vi "LED_control.vi"() -> ()   [LabVIEW 2018]
uses:
  <instrlib>/niDMM/nidmm.llb/niDMM Function.ctl
  <instrlib>/niDMM/nidmm.llb/niDMM Resolution in Digits.ctl
  <instrlib>/niDCPower/nidcpower.llb/niDCPower Measurement Type.ctl
  <instrlib>/niDMM/nidmm.llb/niDMM Configure Measurement Digits.vi
  <vilib>/Instr/_visa.llb/VISA Configure Serial Port (Instr).vi
panel:
  in  "Command":string="led_on"
  in  "Записать":bool
  in  "Tab Control":enum32{"Рабочая область", "Служебная область"}(tab)
  out "Тип индикатора":string
  in  "Питание":bool
  in  "Стоп":bool
  in  "Resource Name":refnum<k15>="PXI1Slot2" caption="Источник питания"
  in  "Мультиметр":refnum<k15>="PXI1Slot3" caption="NI DMM 1"
  in  "V_MB, V":dbl=6.0 caption="voltage level" format="%_6p"
  in  "curlim_V_MB, A":dbl=0.3 caption="current limit" format="%_6p"
  in  "curlim_V_RESERVE, A":dbl=0.1 caption="current limit" format="%_6p"
  out "currentmes_V_MB, A":dbl caption="measurement" format="%_6g"
  out "currentmes_V_RESERVE, A":dbl caption="measurement" format="%_6g"
  in  "V_RESERVE, V":dbl caption="voltage level" format="%_6p"
  out "chart_2":dbl(graph)=8.556104343922883e-07
  out "chart_0":dbl(graph)=5.42616690347781e-05 caption="Waveform Chart 5"
  in  "curlim_V_LED, A":dbl=0.01999999999999985 caption="current limit" format="%_6p"
  in  "V_LED, V":dbl=1.7000000000000006 caption="voltage level" format="%_6p"
  out "chart_1":dbl(graph)=2.456762028615791e-06 caption="Waveform Chart 5"
  out "currentmes_V_LED, A":dbl caption="measurement" format="%_6g"
  in  "NI DMM 1 Current Range 3":string(combo)="0,1" caption="Range"
  out "Real Current, А":dbl=1.3612861948786303e-08 format="%.5f"
  in  "NI DMM 1 units 3":string(combo)="1000" caption="Units"
  out "NI DMM 1 Current Char 3":dbl(graph)=0.013612861948786303
  out "NI DMM 1 Current 3":dbl caption="Current" format="%_6g"
  in  "Arduino":refnum<visa-resource-name>="COM5"
  in  "Сегменты":bool[](array[boolean])=[FALSE, FALSE, FALSE, FALSE, FALSE, FALSE, FALSE, FALSE, FALSE, FALSE]
  out "Разряд":dbl
  out "+/-":bool
  out "Power off":bool
  # "необходимо выдерживать 1 с между нажатиями кнопок"
  # "a"
  # "b"
  # "c"
  # "d"
  # "e"
  # "f"
  # "g"
  # "dp"
  # "all_off - 0\nall_on - 1"
  # "регклировка суммарного тока через инлдикатор"
  # "автоматизировать подбор напряжения по известному максимальному напряжению и току. ОС по току сегмента"
  # "\"опрашивать кнопки не чаще, чем раз в секунду. сейчас кликать можно чаще, они загорятся, но ничего не произойдет\""
  # "регулировать ток в зависимости от температуры.\nс ростом температуры растет ток.\nпид-регулятор??"
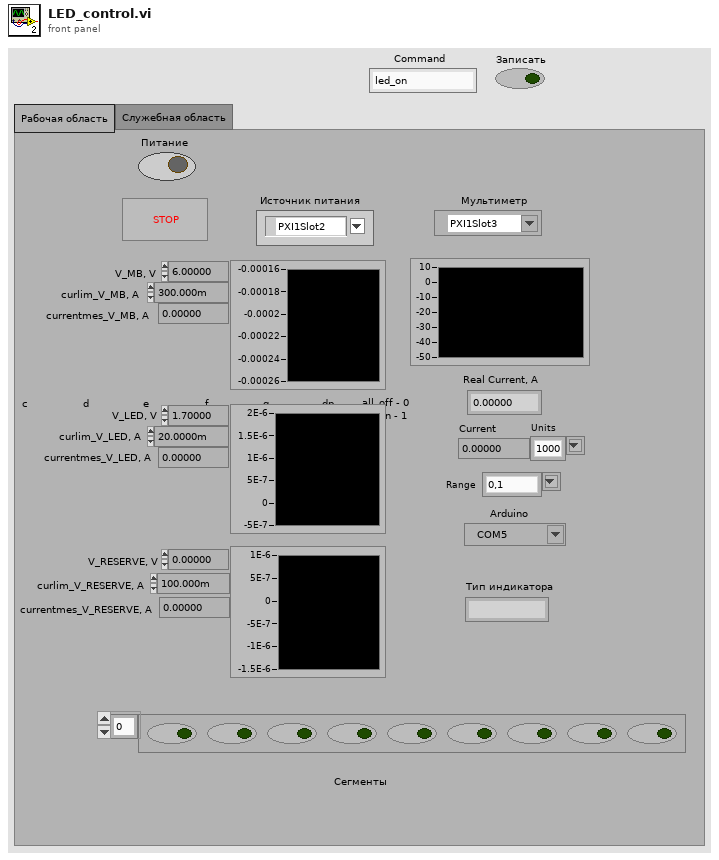
[diagram p1: front panel]
types:
  T1 = typedef "niDMM Function.ctl" = enum16{"DC Volts", "AC Volts", "DC Current", "AC Current", "2-wire Resistance", "4-wire Resistance", "Diode", "Frequency", "Period", "AC Volts DC Coupled", "Capacitance", "Inductance", "Temperature"}
  T2 = typedef "niDMM Resolution in Digits.ctl" = dbl
  T3 = typedef "niDCPower Measurement Type.ctl" = i32
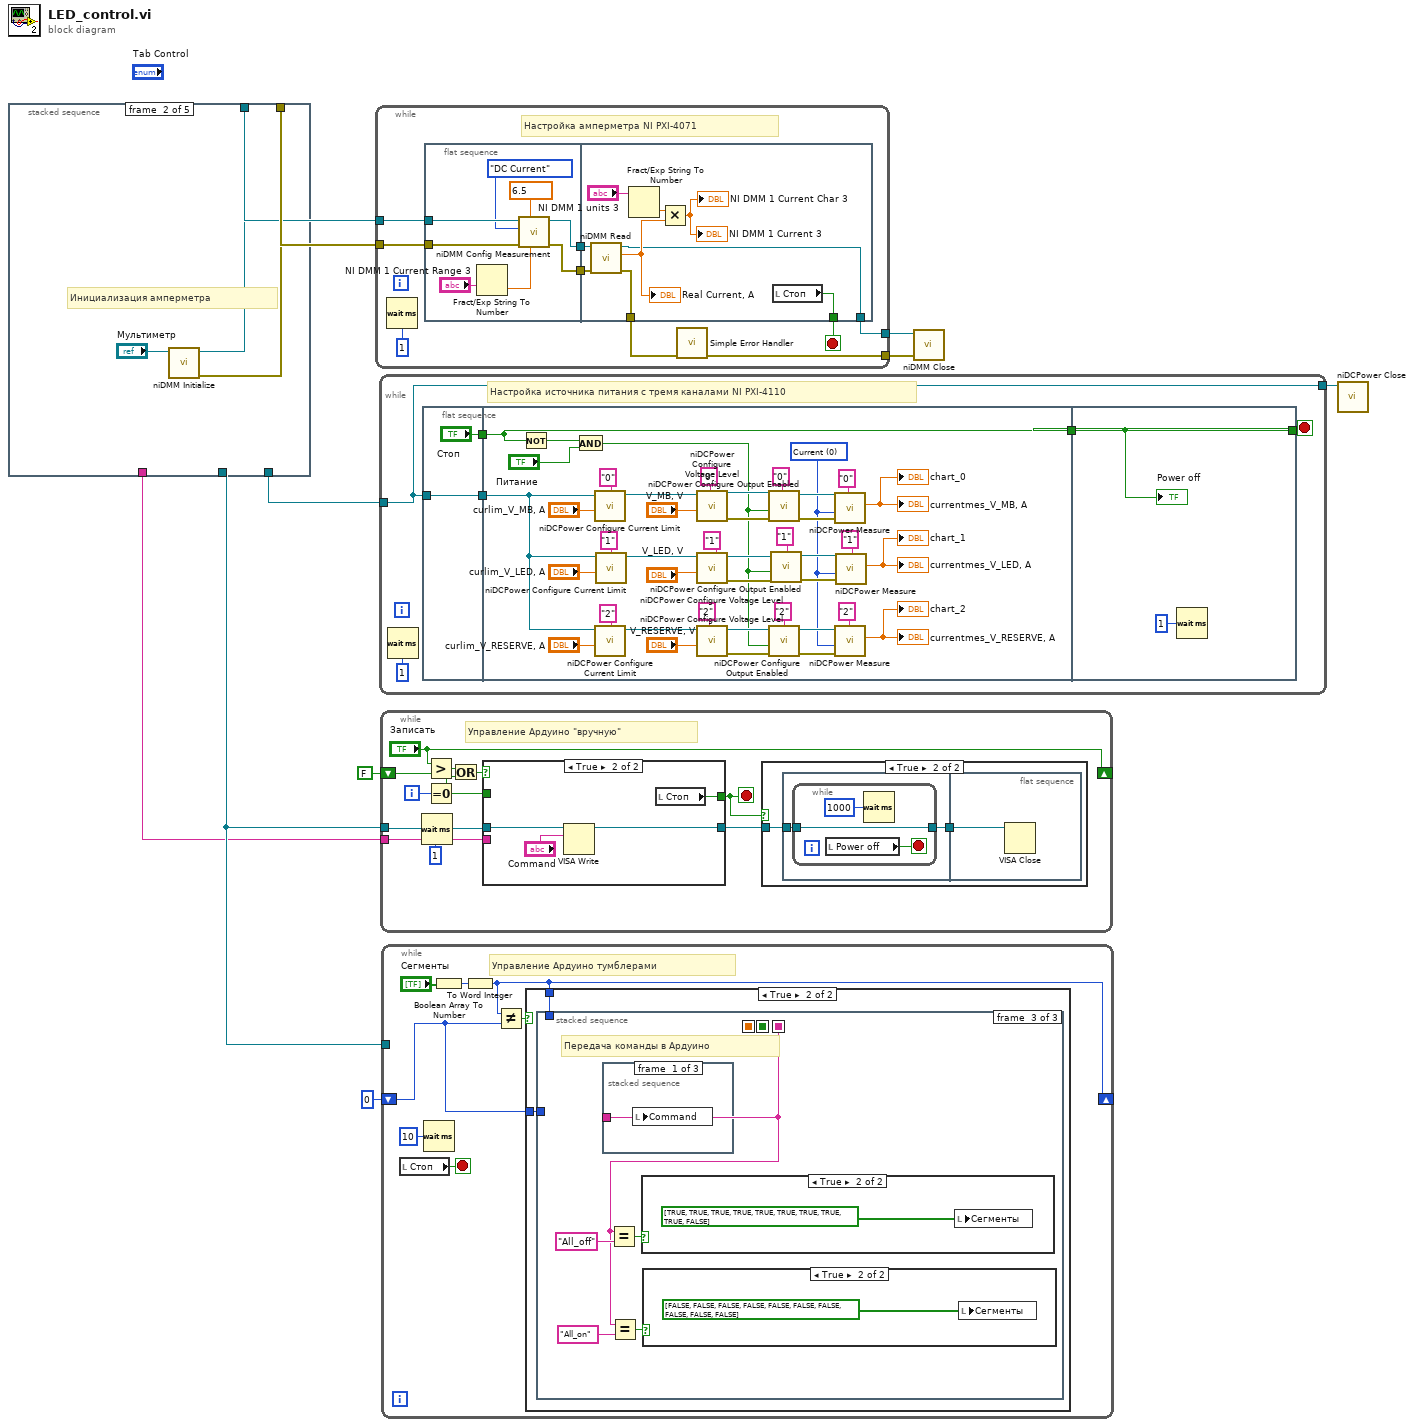
[diagram p0: block diagram]
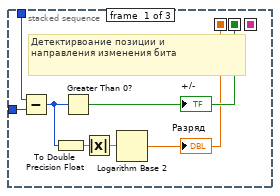
[diagram p3: hidden frame]
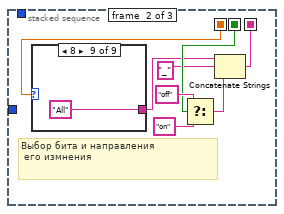
[diagram p4: hidden frame]
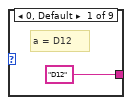
[diagram p5: hidden frame]
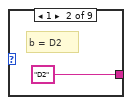
[diagram p6: hidden frame]
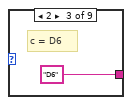
[diagram p7: hidden frame]
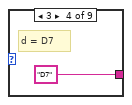
[diagram p8: hidden frame]
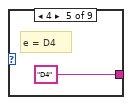
[diagram p9: hidden frame]
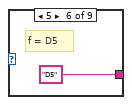
[diagram p10: hidden frame]
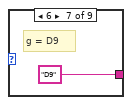
[diagram p11: hidden frame]
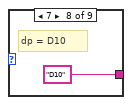
[diagram p12: hidden frame]
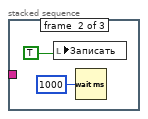
[diagram p15: hidden frame]
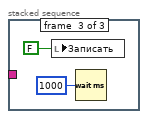
[diagram p16: hidden frame]
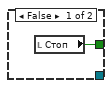
[diagram p18: hidden frame]
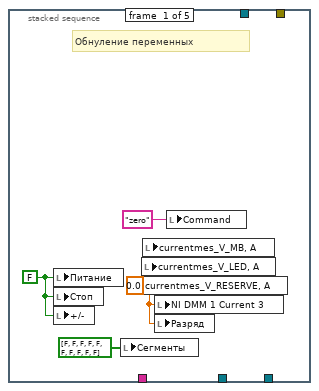
[diagram p19: hidden frame]
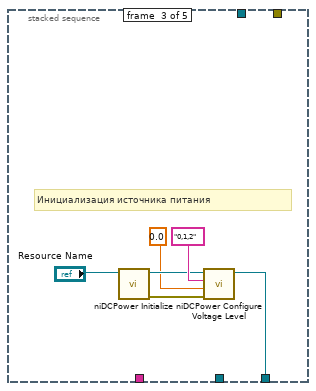
[diagram p20: hidden frame]
diagram:
  n1 = stacked-sequence {
    tunnel: [_ _ w20 _ _] -> w7
    tunnel: [_ w16 _ _ _] -> w10
    tunnel: [_ w15 _ _ _] -> w9
    tunnel: [_ _ _ w24 _] -> w4
    tunnel: [_ _ _ _ w27] -> w1
    frame #0 {
      w13 = 0.0 ("currentmes_2")
      w11 = FALSE ("Стоп")
      # "Обнуление переменных"
      n2 = local write "Питание"(w11) -> ()
      n3 = local write "Стоп"(w11) -> ()
      n4 = local write "+/-"(w11) -> ()
      n5 = local write "Сегменты"(bool[] [FALSE, FALSE, FALSE, FALSE, FALSE, FALSE, FALSE, FALSE, FALSE, FALSE] ("Сегменты")) -> ()
      n6 = local write "currentmes_V_RESERVE, A"(w13) -> ()
      n7 = local write "currentmes_V_LED, A"(w13) -> ()
      n8 = local write "currentmes_V_MB, A"(w13) -> ()
      n9 = local write "NI DMM 1 Current 3"(w13) -> ()
      n10 = local write "Разряд"(w13) -> ()
      n11 = local write "Command"("zero" ("Command 2")) -> ()
    }
    frame #1 {
      # "Инициализация амперметра"
      n12 = call <instrlib>:"niDMM Initialize.vi"("Instrument Descriptor"="Мультиметр") -> ("error out"=w16:errorcluster, "instrument handle out"=w15:refnum<k15>)  [unwired: 9 in]
    }
    frame #2 {
      # "Инициализация источника питания"
      n13 = call <instrlib>:"niDCPower Initialize.vi"("resource name"="Resource Name") -> ("error out"=w19:errorcluster, "instrument handle out"=w21:refnum<k15>)  [unwired: 3 in, 6 out]
      n14 = call <instrlib>:"niDCPower Configure Voltage Level.vi"("error in (no error)"=w19, "voltage level"=0.0, "channel name"="0,1,2", "instrument handle"=w21) -> ("instrument handle out"=w20:refnum<k15>)  [unwired: 6 in, 1 out]
    }
    frame #3 {
      # "Инициализация Ардуино"
      n15 = call-poly "VISA Configure Serial Port"("VISA resource name"="Arduino", "baud rate (9600)"=u32 9600) -> ("VISA resource name out"=w24:refnum<visa-resource-name>)  [unwired: 12 in, 1 out]
    }
    frame #4 {
      # "Всплывающее окно\nкакой индикатор?\nОА/ОК"
      n16 = call "Begin.vi"() -> ("String"=w27:string)  [unwired: 8 in]
      "Тип индикатора" <- w27
      n17 = local write "Command"(w27) -> ()
    }
  }
  n18 = while {
    tunnel: [w34] -> w2
    tunnel: w9 -> [w32]
    tunnel: w10 -> [w31]
    tunnel: [w28] -> w3
    stop <- w30 stop-if-true
    # "Настройка амперметра NI PXI-4071"
    n19 = Wait (ms)(milliseconds to wait=u32 1) -> ()  [unwired: 1 out]
    n20 = flat-sequence {
      tunnel: [w41] -> w36
      tunnel: w32 -> [w39]
      tunnel: w31 -> [w43]
      tunnel: [w40] -> w35
      tunnel: w36 -> [w49]
      tunnel: w35 -> [w52]
      tunnel: [w47] -> w30
      tunnel: [w46] -> w28
      tunnel: [w45] -> w29
      frame #0 {
        w37 = T2 6.5 items=["3 1/2"=3.5, "4 1/2"=4.5, "5 1/2"=5.5, "6 1/2"=6.5, "7 1/2"=7.5] ("Resolution in Digits")
        n21 = Fract/Exp String To Number(string="NI DMM 1 Current Range 3") -> (number=w42:dbl)  [unwired: 3 in, 1 out]
        n22 = call-poly <instrlib>:"niDMM Config Measurement.vi"("Range"=w42, "Resolution in Digits"=w37, "error in (no error)"=w43, "Function"=niDMM_Function."DC Current" ("Measurement Type"), "instrument handle"=w39) -> ("error out"=w40:errorcluster, "instrument handle out"=w41:refnum<k15>)  [unwired: 5 in]
      }
      frame #1 {
        n23 = call <instrlib>:"niDMM Read.vi"("error in (no error)"=w52, "instrument handle"=w49) -> ("error out"=w45:errorcluster, "Measurement"=w48:dbl, "instrument handle out"=w46:refnum<k15>)  [unwired: 7 in]
        "Real Current, А" <- w48
        n24 = Fract/Exp String To Number(string="NI DMM 1 units 3") -> (number=w50:dbl)  [unwired: 3 in, 1 out]
        n25 = Multiply(x=w50, y=w48) -> (x*y=→"NI DMM 1 Current 3" →"NI DMM 1 Current Char 3":dbl)
        n26 = local read "Стоп"() -> (w47:bool)
      }
    }
    n27 = call <vilib>:"Simple Error Handler.vi"("error in (no error)"=w29) -> ("error out"=w34:errorcluster)  [unwired: 1 in, 7 out]
  }
  n28 = while {
    tunnel: w7 -> [w55]
    tunnel: [w55] -> w6
    stop <- w56 stop-if-true
    # "Настройка источника питания с тремя каналами NI PXI-4110"
    n29 = Wait (ms)(milliseconds to wait=u32 1) -> ()  [unwired: 1 out]
    n30 = flat-sequence {
      tunnel: w55 -> [w61]
      tunnel: [w61] -> w58
      tunnel: ["Стоп"] -> w57
      tunnel: w58 -> [w69]
      tunnel: w57 -> [w103]
      tunnel: [w103] -> w54
      tunnel: [w105] -> w56
      tunnel: w54 -> [w105]
      frame #0 {
      }
      frame #1 {
        w68 = T3 0 items=["Current", "Voltage"] ("measurement type")
        n31 = Not(x=w103) -> (.not. x?=w102:bool)
        n32 = And(x=w102, y="Питание") -> (x .and. y?=w64:bool)
        n33 = call <instrlib>:"niDCPower Configure Current Limit.vi"("current limit"="curlim_V_MB, A", "channel name"="0", "instrument handle"=w69) -> ("instrument handle out"=w88:refnum<k15>)  [unwired: 7 in, 1 out]
        n34 = call <instrlib>:"niDCPower Configure Current Limit.vi"("current limit"="curlim_V_RESERVE, A", "channel name"="2", "instrument handle"=w69) -> ("instrument handle out"=w87:refnum<k15>)  [unwired: 7 in, 1 out]
        n35 = call <instrlib>:"niDCPower Configure Current Limit.vi"("current limit"="curlim_V_LED, A", "channel name"="1", "instrument handle"=w69) -> ("instrument handle out"=w96:refnum<k15>)  [unwired: 7 in, 1 out]
        n36 = call <instrlib>:"niDCPower Configure Voltage Level.vi"("voltage level"="V_MB, V", "channel name"="0", "instrument handle"=w88) -> ("error out"=w93:errorcluster, "instrument handle out"=w90:refnum<k15>)  [unwired: 7 in]
        n37 = call <instrlib>:"niDCPower Configure Voltage Level.vi"("voltage level"="V_LED, V", "channel name"="1", "instrument handle"=w96) -> ("error out"=w99:errorcluster, "instrument handle out"=w97:refnum<k15>)  [unwired: 7 in]
        n38 = call <instrlib>:"niDCPower Configure Voltage Level.vi"("voltage level"="V_RESERVE, V", "channel name"="2", "instrument handle"=w87) -> ("error out"=w92:errorcluster, "instrument handle out"=w91:refnum<k15>)  [unwired: 7 in]
        n39 = call <instrlib>:"niDCPower Configure Output Enabled.vi"("error in (no error)"=w93, "output enabled"=w64, "channel name"="0", "instrument handle"=w90) -> ("error out"=w83:errorcluster, "instrument handle out"=w84:refnum<k15>)  [unwired: 6 in]
        n40 = call <instrlib>:"niDCPower Configure Output Enabled.vi"("error in (no error)"=w92, "output enabled"=w64, "channel name"="2", "instrument handle"=w91) -> ("error out"=w82:errorcluster, "instrument handle out"=w81:refnum<k15>)  [unwired: 6 in]
        n41 = call <instrlib>:"niDCPower Configure Output Enabled.vi"("error in (no error)"=w99, "output enabled"=w64, "channel name"="1", "instrument handle"=w97) -> ("error out"=w100:errorcluster, "instrument handle out"=w98:refnum<k15>)  [unwired: 6 in]
        n42 = call <instrlib>:"niDCPower Measure.vi"("error in (no error)"=w83, "measurement type"=w68, "channel name"="0", "instrument handle"=w84) -> ("measurement"=→"currentmes_V_MB, A" →"chart_0":dbl)  [unwired: 5 in, 2 out]
        n43 = call <instrlib>:"niDCPower Measure.vi"("error in (no error)"=w82, "measurement type"=w68, "channel name"="2", "instrument handle"=w81) -> ("measurement"=→"currentmes_V_RESERVE, A" →"chart_2":dbl)  [unwired: 5 in, 2 out]
        n44 = call <instrlib>:"niDCPower Measure.vi"("error in (no error)"=w100, "measurement type"=w68, "channel name"="1", "instrument handle"=w98) -> ("measurement"=→"chart_1" →"currentmes_V_LED, A":dbl)  [unwired: 5 in, 2 out]
      }
      frame #2 {
        n45 = Wait (ms)(milliseconds to wait=u32 1) -> ()  [unwired: 1 out]
        "Power off" <- w105
      }
    }
  }
  n46 = while {
    tunnel: w4 -> [w113]
    shift-right: ["Записать"] -> _
    shift-left: FALSE ("Записать") -> [w115]
    tunnel: w1 -> [w111]
    i -> [w112]
    stop <- w107 stop-if-true
    # "Управление Ардуино \"вручную\""
    n47 = Wait (ms)(milliseconds to wait=u32 1) -> ()  [unwired: 1 out]
    n48 = Greater?(x="Записать", y=w115) -> (0:w109:bool)
    n49 = Equal To 0?(x=w112) -> (x = 0?=w108:bool)
    n50 = Or(x=w109, y=w108) -> (x .or. y?=w110:bool)
    n51 = case shown="True" w110 {
      tunnel: w113 -> [_ w129]
      tunnel: [w125 w128] -> w107
      tunnel: w111 -> [_ _]
      tunnel: w108 -> [_ _]
      tunnel: [_ w126] -> w106
      frame False {
        n52 = local read "Стоп"() -> (w125:bool)
      }
      frame True {
        n53 = VISA Write(VISA resource name=w129, write buffer="Command") -> (VISA resource name out=w126:refnum<visa-resource-name>)  [unwired: 1 in, 2 out]
        n54 = local read "Стоп"() -> (w128:bool)
      }
    }
    n55 = case shown="True" w107 {
      tunnel: w106 -> [_ w118]
      frame False {
      }
      frame True {
        n56 = flat-sequence {
          tunnel: w118 -> [w120]
          tunnel: [w119] -> w117
          tunnel: w117 -> [w124]
          frame #0 {
            n57 = while {
              tunnel: w120 -> [w121]
              tunnel: [w121] -> w119
              stop <- w122 stop-if-true
              n58 = local read "Power off"() -> (w122:bool)
              n59 = Wait (ms)(milliseconds to wait=u32 1000) -> ()  [unwired: 1 out]
            }
          }
          frame #1 {
            n60 = VISA Close(VISA resource name=w124) -> ()  [unwired: 1 in, 1 out]
          }
        }
      }
    }
  }
  n61 = while {
    shift-right: [w130] -> _
    shift-left: i16 0 -> [w132]
    tunnel: w4 -> [_]
    stop <- w136 stop-if-true
    # "Управление Ардуино тумблерами"
    n62 = local read "Стоп"() -> (w136:bool)
    n63 = Wait (ms)(milliseconds to wait=u32 10 ("millisecond timer value")) -> ()  [unwired: 1 out]
    n64 = Boolean Array To Number(Boolean array="Сегменты") -> (number=w131:u32)
    n65 = To Word Integer(number=w131) -> (16bit integer=w130:i16)
    n66 = Not Equal?(x=w130, y=w132) -> (x != y?=w133:bool)
    n67 = case shown="True" w133 {
      tunnel: w130 -> [_ w137]
      tunnel: w132 -> [_ w138]
      frame False {
      }
      frame True {
        n68 = stacked-sequence {
          seq-local: [w141 _ _] -> [_ w151 _]
          seq-local: [w139 _ _] -> [_ w146 _]
          seq-local: [_ w147 _] -> [_ _ w164]
          tunnel: w137 -> [w143 _ _]
          tunnel: w138 -> [w142 _ _]
          frame #0 {
            # "Детектирвоание позиции и\nнаправления изменения бита"
            n69 = Subtract(x=w143, y=w142) -> (x-y=w144:i16)
            n70 = To Double Precision Float(number=w144) -> (double precision float=w145:dbl)
            n71 = Greater Than 0?(x=w144) -> (x > 0?=w141:bool)
            "+/-" <- w141
            n72 = Absolute Value(x=w145) -> (abs(x)=w140:dbl)
            n73 = Logarithm Base 2(1:w140) -> (0:w139:dbl)
            "Разряд" <- w139
          }
          frame #1 {
            # "Выбор бита и направления\n его измнения"
            n74 = case shown="8" w146 {
              tunnel: ["D12" "D2" "D6" "D7" "D4" "D5" "D9" "D10" "All"] -> w149
              frame 0, Default {
                # "a = D12"
              }
              frame 1 {
                # "b = D2"
              }
              frame 2 {
                # "c = D6"
              }
              frame 3 {
                # "d = D7"
              }
              frame 4 {
                # "e = D4"
              }
              frame 5 {
                # "f = D5"
              }
              frame 6 {
                # "g = D9"
              }
              frame 7 {
                # "dp = D10"
              }
              frame 8 {
              }
            }
            n75 = Select(t="off", s=w151, f="on") -> (s? t:f=w148:string)
            n76 = Concatenate Strings(w149, "_" ("string"), w148) -> (w147:string)
          }
          frame #2 {
            # "Передача команды в Ардуино"
            n77 = stacked-sequence {
              tunnel: w164 -> [w170 _ _]
              frame #0 {
                n78 = local write "Command"(w170) -> ()
              }
              frame #1 {
                n79 = local write "Записать"(TRUE ("Записать")) -> ()
                n80 = Wait (ms)(milliseconds to wait=u32 1000) -> ()  [unwired: 1 out]
              }
              frame #2 {
                n81 = local write "Записать"(FALSE ("Записать")) -> ()
                n82 = Wait (ms)(milliseconds to wait=u32 1000) -> ()  [unwired: 1 out]
              }
            }
            n83 = Equal?(x=w164, y="All_off") -> (x = y?=w167:bool)
            n84 = Equal?(x=w164, y="All_on") -> (x = y?=w165:bool)
            n85 = case shown="True" w167 {
              frame False {
              }
              frame True {
                n86 = local write "Сегменты"(bool[] [TRUE, TRUE, TRUE, TRUE, TRUE, TRUE, TRUE, TRUE, TRUE, FALSE] ("Сегменты")) -> ()
              }
            }
            n87 = case shown="True" w165 {
              frame False {
              }
              frame True {
                n88 = local write "Сегменты"(bool[] [FALSE, FALSE, FALSE, FALSE, FALSE, FALSE, FALSE, FALSE, FALSE, FALSE] ("Сегменты")) -> ()
              }
            }
          }
        }
      }
    }
  }
  n89 = call <instrlib>:"niDMM Close.vi"("error in (no error)"=w2, "instrument handle"=w3) -> ()  [unwired: 9 in, 1 out]
  n90 = call <instrlib>:"niDCPower Close.vi"("instrument handle"=w6) -> ()  [unwired: 10 in, 1 out]
